vi "Save Projects and Libraries.vi"(8 "error in (no error)":errorcluster) -> (0 "error out":errorcluster)   [LabVIEW 2021, in "Migrator.lvlib"]
uses:
  Migrator.lvlib
  Migrator Reusables/Migrator Reusables.lvlib
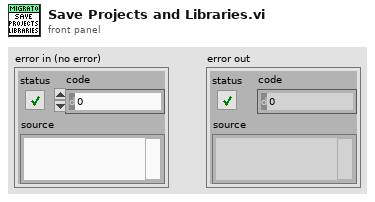
[diagram p1: front panel]
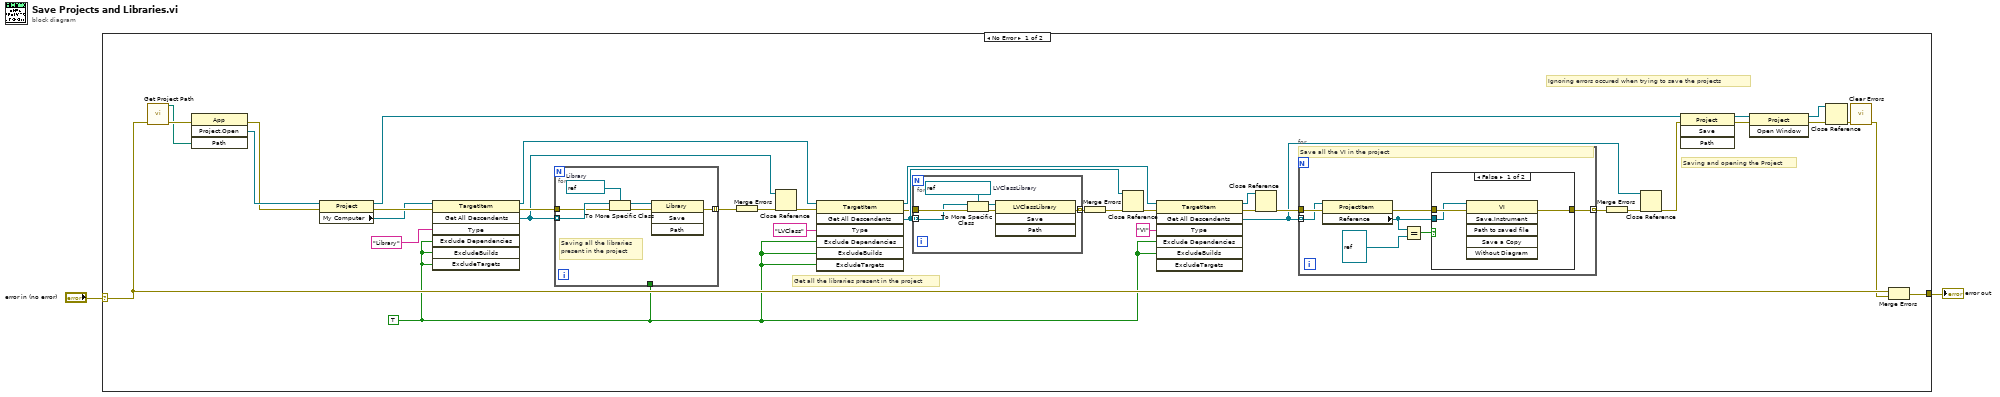
[diagram p0: block diagram]
diagram:
  n1 = case shown="No Error" "error in (no error)" {
    selector: "error in (no error)" -> [w31 w64]
    tunnel: [w32 w64] -> w2
    frame No Error {
      w7 = TRUE ("ExcludeDependencies")
      # "Get all the libraries present in the project"
      # "Saving and opening the Project"
      # "Ignoring errors occured when trying to save the projects"
      n2 = call "Get Project Path.vi"("error in (no error)"=w31) -> ("Project Path Out"=w39:path, "error out"=w40:errorcluster)  [unwired: 13 in]
      n3 = invoke class="App" method="Project.Open"(error in=w40, "Path"=w39) -> (error out=w34:errorcluster, "Project:Open"=w36:refnum<vi>)  [unwired: 2 in, 2 out]
      n4 = property class="Project"(reference=w36, error in=w34) -> (reference out=w30:refnum<vi>, error out=w20:errorcluster, "My Computer"=w19:refnum<vi>)
      n5 = invoke class="TargetItem" method="Get All Descendents"(reference=w19, error in=w20, "Type"="Library", "Exclude Dependencies"=w7, "ExcludeBuilds"=w7, "ExcludeTargets"=w7) -> (reference out=w21:refnum<vi>, error out=w38:errorcluster, "All Descendents"=w28:refnum<vi>[])  [unwired: 1 in, 4 out]
      n6 = for {
        tunnel: w28 -> [w46] mode=indexing
        tunnel: w38 -> [w43]
        tunnel: [w44] -> w35 mode=indexing
        tunnel: w7 -> [_]
        w45 = refnum<vi> refnum  # Library
        # "Saving all the libraries \npresent in the project"
        n7 = To More Specific Class(target class=w45, reference=w46, error in=w43) -> (specific class reference=w42:refnum<vi>, error out=w41:errorcluster)
        n8 = invoke class="Library" method="Save"(reference=w42, error in=w41) -> (error out=w44:errorcluster)  [unwired: 2 in, 3 out]
      }
      n9 = Merge Errors(w35) -> (w29:errorcluster)
      n10 = Close Reference(reference=w28, error in (no error)=w29) -> (error out=w22:errorcluster)
      n11 = invoke class="TargetItem" method="Get All Descendents"(reference=w21, error in=w22, "Type"="LVClass", "Exclude Dependencies"=w7, "ExcludeBuilds"=w7, "ExcludeTargets"=w7) -> (reference out=w14:refnum<vi>, error out=w23:errorcluster, "All Descendents"=w27:refnum<vi>[])  [unwired: 1 in, 4 out]
      n12 = for {
        tunnel: w27 -> [w58] mode=indexing
        tunnel: w23 -> [w60]
        tunnel: [w61] -> w25 mode=indexing
        w63 = refnum<vi> refnum  # LVClassLibrary
        n13 = To More Specific Class(target class=w63, reference=w58, error in=w60) -> (specific class reference=w62:refnum<vi>, error out=w59:errorcluster)
        n14 = invoke class="LVClassLibrary" method="Save"(reference=w62, error in=w59) -> (error out=w61:errorcluster)  [unwired: 2 in, 3 out]
      }
      n15 = Merge Errors(w25) -> (w26:errorcluster)
      n16 = Close Reference(reference=w27, error in (no error)=w26) -> (error out=w13:errorcluster)
      n17 = invoke class="TargetItem" method="Get All Descendents"(reference=w14, error in=w13, "Type"="VI", "Exclude Dependencies"=w7, "ExcludeBuilds"=w7) -> (reference out=w16:refnum<vi>, error out=w17:errorcluster, "All Descendents"=w8:refnum<vi>[])  [unwired: 2 in, 4 out]
      n18 = Close Reference(reference=w16, error in (no error)=w17) -> (error out=w15:errorcluster)
      n19 = for {
        tunnel: w8 -> [w47] mode=indexing
        tunnel: w15 -> [w49]
        tunnel: [w48] -> w11 mode=indexing
        # "Save all the VI in the project"
        n20 = property class="ProjectItem"(reference=w47, error in=w49) -> (error out=w53:errorcluster, "Reference"=w50:refnum<vi>)  [unwired: 1 out]
        n21 = Equal?(x=w50, y=refnum<vi> refnum) -> (x = y?=w51:bool)
        n22 = case shown="False" w51 {
          tunnel: [w54 w57] -> w48
          tunnel: w53 -> [w56 w57]
          tunnel: w50 -> [w55 _]
          frame False {
            n23 = invoke class="VI" method="Save.Instrument"(reference=w55, error in=w56) -> (error out=w54:errorcluster)  [unwired: 4 in, 5 out]
          }
          frame True {
          }
        }
      }
      n24 = Merge Errors(w11) -> (w10:errorcluster)
      n25 = Close Reference(reference=w8, error in (no error)=w10) -> (error out=w9:errorcluster)
      n26 = invoke class="Project" method="Save"(reference=w30, error in=w9) -> (reference out=w4:refnum<vi>, error out=w6:errorcluster)  [unwired: 2 in, 2 out]
      n27 = invoke class="Project" method="Open Window"(reference=w4, error in=w6) -> (reference out=w3:refnum<vi>, error out=w5:errorcluster)  [unwired: 1 in, 1 out]
      n28 = Close Reference(reference=w3, error in (no error)=w5) -> (error out=w33:errorcluster)
      n29 = call <vilib>:"Clear Errors.vi"("error in (no error)"=w33) -> ("error out"=w18:errorcluster)  [unwired: 5 in, 1 out]
      n30 = Merge Errors(w31, w18) -> (w32:errorcluster)
    }
    frame Error {
    }
  }
  "error out" <- w2
